vi "Process Bookmarks.vi"(8 "error in (no error)":errorcluster {"code" format="Error %.0f"}, 10 "Bookmarked Map":T1(c390), 11 "VIDoc Printer In":refnum<class "VIDoc Printer.lvclass">) -> (0 "error out":errorcluster {"code" format="Error %.0f"}, 3 "VIDoc Printer Out":refnum<class "VIDoc Printer.lvclass">)   [LabVIEW 2023, in "VIDoc Printer.lvlib" / "VIDoc Printer.lvclass"]
uses:
  VIDoc Printer.lvclass
  VIDoc Printer.lvclass/VIDoc Printer.ctl
  Parsing/GUI Documentation/GUI Documentation.lvclass
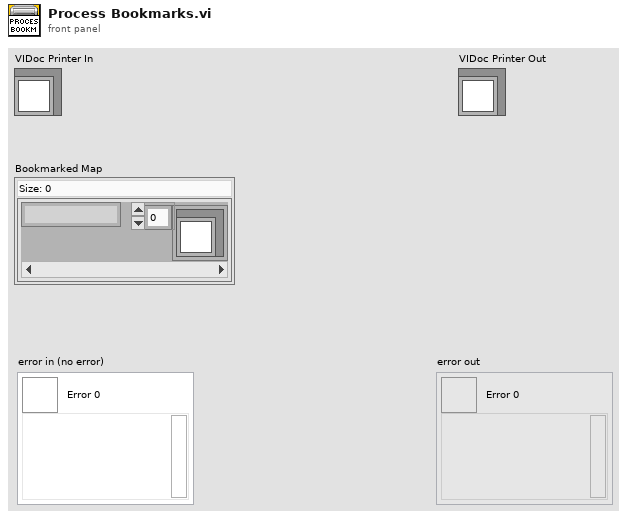
[diagram p1: front panel]
types:
  T1 = map{string, refnum<class "GUI Documentation.lvclass">[]}
  T2 = typedef "VIDoc Printer.lvlib/VIDoc Printer.lvclass/Process VI Enum.ctl" = enum16{"Header", "Memory", "By Folder", "By Tree", "By List", "Method Details", "FP"}
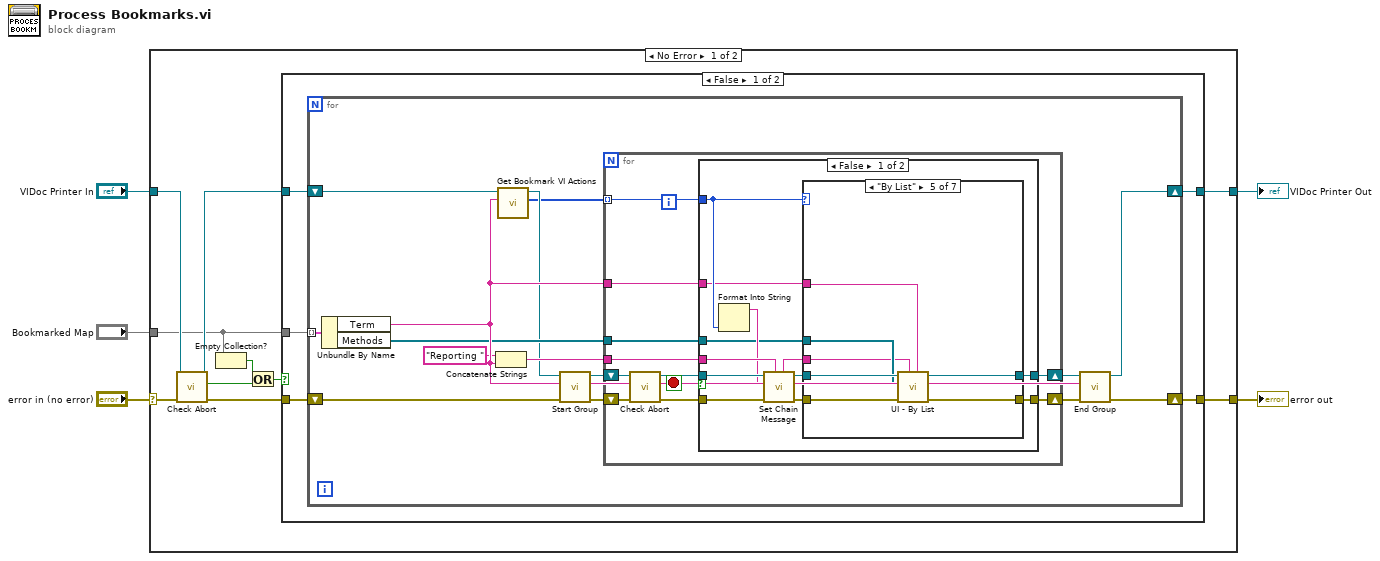
[diagram p0: block diagram]
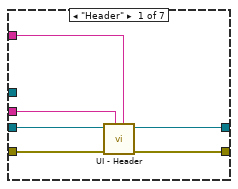
[diagram p2: hidden frame]
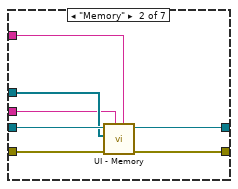
[diagram p3: hidden frame]
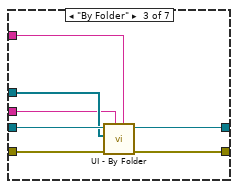
[diagram p4: hidden frame]
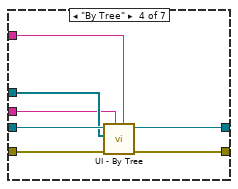
[diagram p5: hidden frame]
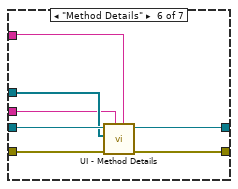
[diagram p6: hidden frame]
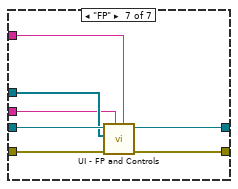
[diagram p7: hidden frame]
diagram:
  n1 = case shown="No Error" "error in (no error)" {
    selector: "error in (no error)" -> [w15 w112]
    tunnel: [w10 w112] -> w4
    tunnel: [w9 w111] -> w2
    tunnel: "VIDoc Printer In" -> [w12 w111]
    tunnel: "Bookmarked Map" -> [w7 _]
    frame No Error {
      n2 = call "Check Abort.vi"("error in (no error)"=w15, "VIDoc Printer In"=w12) -> ("error out"=w14:errorcluster, "Abort?"=w11:bool, "VIDoc Printer Out"=w13:refnum<class "VIDoc Printer.lvclass">)  [unwired: 7 in]
      n3 = Empty Collection?(1:w7) -> (0:w6:bool)
      n4 = Or(x=w6, y=w11) -> (x .or. y?=w8:bool)
      n5 = case shown="False" w8 {
        tunnel: w14 -> [w20 w110]
        tunnel: w13 -> [w17 w109]
        tunnel: [w18 w110] -> w10
        tunnel: [w19 w109] -> w9
        tunnel: w7 -> [w16 _]
        frame False {
          n6 = for {
            shift-right: [w33] -> w18
            shift-left: w20 -> [w35]
            shift-right: [w34] -> w19
            shift-left: w17 -> [w32]
            tunnel: w16 -> [w31] mode=indexing
            n7 = Unbundle By Name(w31) -> ("Term"=w30:string, "Methods"=w29:refnum<class "GUI Documentation.lvclass">[])
            n8 = Concatenate Strings("Reporting " ("string"), w30) -> (w27:string)
            n9 = call "Get Bookmark VI Actions.vi"("Term"=w30, "VIDoc Printer In"=w32) -> ("Bookmark VI Actions"=w21:T2[], "VIDoc Printer Out"=w22:refnum<class "VIDoc Printer.lvclass">)  [unwired: 7 in, 1 out]
            n10 = call-dynamic "Start Group.vi"("error in (no error)"=w35, "Group"=w30, "VIDoc Printer In"=w22) -> ("error out"=w26:errorcluster, "VIDoc Printer Out"=w25:refnum<class "VIDoc Printer.lvclass">)  [unwired: 7 in]
            n11 = for {
              shift-right: [w44] -> w23
              shift-left: w26 -> [w46]
              tunnel: w27 -> [w40]
              tunnel: w29 -> [w39]
              shift-right: [w42] -> w24
              shift-left: w25 -> [w45]
              tunnel: w21 -> [w38] mode=indexing
              tunnel: w30 -> [w36]
              stop <- w37 stop-if-true
              n12 = call "Check Abort.vi"("error in (no error)"=w46, "VIDoc Printer In"=w45) -> ("error out"=w43:errorcluster, "Abort?"=w37:bool, "VIDoc Printer Out"=w41:refnum<class "VIDoc Printer.lvclass">)  [unwired: 7 in]
              n13 = case shown="False" w37 {
                tunnel: [w58 w108] -> w44
                tunnel: w43 -> [w55 w108]
                tunnel: [w57 w107] -> w42
                tunnel: w41 -> [w53 w107]
                tunnel: w40 -> [w52 _]
                tunnel: w39 -> [w49 _]
                tunnel: w38 -> [w51 _]
                tunnel: w36 -> [w47 _]
                frame False {
                  n14 = Format Into String(w51) -> (resulting string=w50:string)  [unwired: 3 in, 1 out]
                  n15 = call "Set Chain Message.vi"("Msg Chain"=w52, "error in (no error)"=w55, "New"=w50, "VIDoc Printer In"=w53) -> ("error out"=w56:errorcluster, "VIDoc Printer Out"=w54:refnum<class "VIDoc Printer.lvclass">, "Msg Chain out"=w48:string)  [unwired: 5 in]
                  n16 = case shown="\"By List\"" w51 {
                    tunnel: w56 -> [w63 w70 w77 w84 w91 w98 w105]
                    tunnel: [w61 w68 w75 w82 w89 w96 w103] -> w58
                    tunnel: w54 -> [w64 w71 w78 w85 w92 w99 w106]
                    tunnel: [w62 w69 w76 w83 w90 w97 w104] -> w57
                    tunnel: w49 -> [_ w67 w74 w81 w88 w95 w102]
                    tunnel: w48 -> [w60 w66 w73 w80 w87 w94 w101]
                    tunnel: w47 -> [w59 w65 w72 w79 w86 w93 w100]
                    frame "Header" {
                      n17 = call-dynamic "UI - Header.vi"("Term (Methods)"=w59, "Msg Chain"=w60, "error in"=w63, "VIDoc Printer In"=w64) -> ("error out"=w61:errorcluster, "VIDoc Printer Out"=w62:refnum<class "VIDoc Printer.lvclass">)  [unwired: 6 in]
                    }
                    frame "Memory" {
                      n18 = call-dynamic "UI - Memory.vi"("Term (Methods)"=w65, "Msg Chain"=w66, "error in (no error)"=w70, "UI Docs"=w67, "VIDoc Printer In"=w71) -> ("error out"=w68:errorcluster, "VIDoc Printer Out"=w69:refnum<class "VIDoc Printer.lvclass">)  [unwired: 5 in]
                    }
                    frame "By Folder" {
                      n19 = call-dynamic "UI - By Folder.vi"("Term (Methods)"=w72, "Msg Chain"=w73, "error in (no error)"=w77, "UI Docs"=w74, "VIDoc Printer In"=w78) -> ("error out"=w75:errorcluster, "VIDoc Printer Out"=w76:refnum<class "VIDoc Printer.lvclass">)  [unwired: 5 in]
                    }
                    frame "By Tree" {
                      n20 = call-dynamic "UI - By Tree.vi"("Term (Methods)"=w79, "Msg Chain"=w80, "error in (no error)"=w84, "UI Docs"=w81, "VIDoc Printer In"=w85) -> ("error out"=w82:errorcluster, "VIDoc Printer Out"=w83:refnum<class "VIDoc Printer.lvclass">)  [unwired: 5 in]
                    }
                    frame "By List" {
                      n21 = call-dynamic "UI - By List.vi"("Term (Methods)"=w86, "Msg Chain"=w87, "error in (no error)"=w91, "UI Docs"=w88, "VIDoc Printer In"=w92) -> ("error out"=w89:errorcluster, "VIDoc Printer Out"=w90:refnum<class "VIDoc Printer.lvclass">)  [unwired: 5 in]
                    }
                    frame "Method Details" {
                      n22 = call-dynamic "UI - Method Details.vi"("Term (Methods)"=w93, "Msg Chain"=w94, "error in (no error)"=w98, "UI Docs"=w95, "VIDoc Printer In"=w99) -> ("error out"=w96:errorcluster, "VIDoc Printer Out"=w97:refnum<class "VIDoc Printer.lvclass">)  [unwired: 5 in]
                    }
                    frame "FP" {
                      n23 = call-dynamic "UI - FP and Controls.vi"("Term (Methods)"=w100, "Msg Chain"=w101, "error in (no error)"=w105, "UI Docs"=w102, "VIDoc Printer In"=w106) -> ("error out"=w103:errorcluster, "VIDoc Printer Out"=w104:refnum<class "VIDoc Printer.lvclass">)  [unwired: 5 in]
                    }
                  }
                }
                frame True {
                }
              }
            }
            n24 = call-dynamic "End Group.vi"("error in (no error)"=w23, "Group"=w30, "VIDoc Printer In"=w24) -> ("error out"=w33:errorcluster, "VIDoc Printer Out"=w34:refnum<class "VIDoc Printer.lvclass">)  [unwired: 7 in]
          }
        }
        frame True {
        }
      }
    }
    frame Error {
    }
  }
  "error out" <- w4
  "VIDoc Printer Out" <- w2
